vi "Write present.vi"(8 "error in (no error)":errorcluster, 10 "present?":bool=TRUE, 11 "Serial IO in":refnum<class "Serial IO.lvclass">) -> (0 "error out":errorcluster, 3 "Serial IO out":refnum<class "Serial IO.lvclass">)   [LabVIEW 2013, in "Serial IO.lvclass"]
uses:
  Serial IO.lvclass
  Serial IO.lvclass/Serial IO.ctl
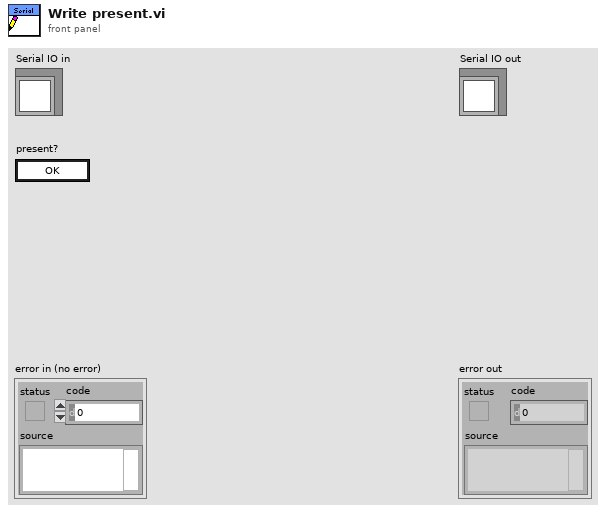
[diagram p1: front panel]
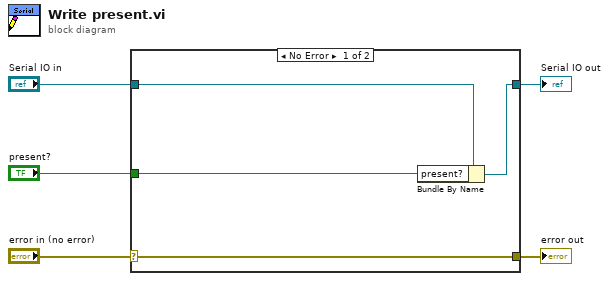
[diagram p0: block diagram]
diagram:
  n1 = case shown="No Error" "error in (no error)" {
    selector: "error in (no error)" -> [w9 w10]
    tunnel: [w9 w10] -> w4
    tunnel: [w7 w11] -> w2
    tunnel: "Serial IO in" -> [w8 w11]
    tunnel: "present?" -> [w6 _]
    frame No Error {
      n2 = Bundle By Name(cluster=w8, "present?"=w6) -> (w7:refnum<class "Serial IO.lvclass">)
    }
    frame Error {
    }
  }
  "error out" <- w4
  "Serial IO out" <- w2
